vi "Register HTTP Handlers.vi"(8 "error in (no error)":errorcluster, 11 "Vecto in":refnum<class "Vecto.lvclass">) -> (0 "error out":errorcluster, 3 "Vecto out":refnum<class "Vecto.lvclass">)   [LabVIEW 2020, in "Vecto.lvlib" / "Vecto.lvclass"]
uses:
  Vecto.lvclass
  InfoController/InfoController.lvclass
  C:/Program Files (x86)/National Instruments/LabVIEW 2024/vi.lib/IlluminatedG/IG HTTP Server/HTTP Server/Handler/Handler.lvclass
  Vecto.lvclass/Vecto.ctl
  VectoService/VectoInfo.lvclass
  C:/Program Files (x86)/National Instruments/LabVIEW 2024/vi.lib/IlluminatedG/IG HTTP Server/HTTP Server/Service/Service.lvclass
  InfoService/NodeStatus.lvclass
  HTTPStatsHandler/HTTPStatsHandler.lvclass
  <vilib>/IlluminatedG/IG HTTP Server/HTTP Server/Server/Add Connection Handler.vi
  <vilib>/IlluminatedG/IG HTTP Server/HTTP Server/Server/Add Request Handler.vi
  <vilib>/IlluminatedG/IG HTTP Server/HTTP Server/Server/Add Route Handler.vi
  <vilib>/IlluminatedG/IG HTTP Server/HTTP Server/Server/Add Controller Handler.vi
  <vilib>/IlluminatedG/IG HTTP Server/HTTP Server/Server/Add Controller.vi
  <vilib>/IlluminatedG/IG HTTP Server/HTTP Server/Server/Add Response Handler.vi
  <vilib>/IlluminatedG/IG HTTP Server/HTTP Server/Server/Add Complete Handler.vi
  <vilib>/IlluminatedG/IG HTTP Server/HTTP Server/Server/Add Exception Handler.vi
  <vilib>/IlluminatedG/IG HTTP Server/HTTP Server/Connection Handler/Connection Handler.lvclass
  <vilib>/IlluminatedG/IG HTTP Server/HTTP Server/Request Handler/Request Handler.lvclass
  <vilib>/IlluminatedG/IG HTTP Server/HTTP Server/Route Handler/Route Handler.lvclass
  <vilib>/IlluminatedG/IG HTTP Server/HTTP Server/Controller Handler/Controller Handler.lvclass
  <vilib>/IlluminatedG/IG HTTP Server/HTTP Server/Controller/Controller.lvclass
  <vilib>/IlluminatedG/IG HTTP Server/HTTP Server/Response Handler/Response Handler.lvclass
  <vilib>/IlluminatedG/IG HTTP Server/HTTP Server/Complete Handler/Complete Handler.lvclass
  <vilib>/IlluminatedG/IG HTTP Server/HTTP Server/Exception Handler/Exception Handler.lvclass
  <vilib>/IlluminatedG/IG HTTP Server/HTTP Server/Handler/Handler.lvclass
  <vilib>/IlluminatedG/IG HTTP Server/HTTP Server/Server/Server.lvclass
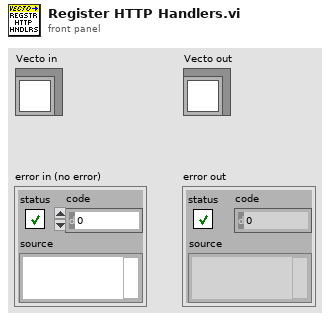
[diagram p1: front panel]
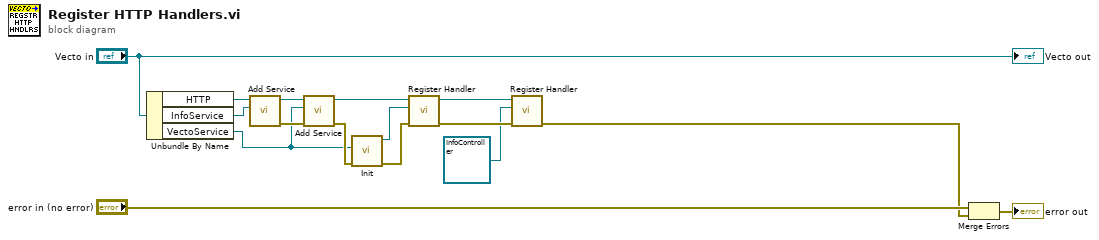
[diagram p0: block diagram]
diagram:
  n1 = Unbundle By Name("Vecto in") -> ("HTTP"=w5:refnum<class "Server.lvclass">, "InfoService"=w4:refnum<class "NodeStatus.lvclass">, "VectoService"=w2:refnum<class "VectoInfo.lvclass">)
  n2 = call <vilib>:"Add Service.vi"("Service"=w4, "Server in"=w5) -> ("error out"=w15:errorcluster, "Server out"=w3:refnum<class "Server.lvclass">)  [unwired: 8 in]
  n3 = call <vilib>:"Add Service.vi"("error in (no error)"=w15, "Service"=w2, "Server in"=w3) -> ("error out"=w16:errorcluster, "Server out"=w1:refnum<class "Server.lvclass">)  [unwired: 7 in]
  n4 = call "Init.vi"("error in (no error)"=w16, "VectoService"=w2) -> ("error out"=w14:errorcluster, "HTTPStatsHandler out"=w13:refnum<class "HTTPStatsHandler.lvclass">)  [unwired: 8 in]
  n5 = call <vilib>:"Register Handler.vi"("error in (no error)"=w14, "Handler"=w13, "Server in"=w1) -> ("error out"=w10:errorcluster, "Server out"=w9:refnum<class "Server.lvclass">)  [unwired: 7 in]
  n6 = call <vilib>:"Register Handler.vi"("error in (no error)"=w10, "Handler"=refnum<class "InfoController.lvclass"> refnum ("Vecto.lvlib:InfoController.lvclass"), "Server in"=w9) -> ("error out"=w7:errorcluster)  [unwired: 7 in, 1 out]
  n7 = Merge Errors("error in (no error)", w7) -> (→"error out":errorcluster)
  "Vecto out" <- "Vecto in"
